vi "Read Lockin Parameters.vi"(0 "tdms file":refnum<k34>, 5 "group name in":string, 9 "Channel name":string, 11 "Error In":errorcluster, 12 "Lockin parameters":T1={"Frequency"=0.0, "Phase"=0.0, "Syncronous"=FALSE, "Points per sine wave"=0, "DDS"=FALSE, "Frequency word"=0, "Phase word"=0, "DDS modulus"=15120, "DDS clock"=125000000.0} {"DDS clock" format="%_17pHz"; "DDS modulus" format="0x%x (%d)"; "Phase" format="%#_gdeg"; "Frequency" format="%_17pHz"}) -> (2 "dt":dbl, 3 "found":bool, 4 "tdms file out":refnum<k34>, 8 "t0":timestamp, 10 "Channel length":u64, 14 "Lockin parameters out":T1={"Frequency"=0.0, "Phase"=0.0, "Syncronous"=FALSE, "Points per sine wave"=0, "DDS"=FALSE, "Frequency word"=0, "Phase word"=0, "DDS modulus"=15120, "DDS clock"=125000000.0} {"DDS clock" format="%_17pHz"; "DDS modulus" format="0x%x (%d)"; "Phase" format="%#_gdeg"; "Frequency" format="%_17pHz"}, 15 "Error Out":errorcluster)   [LabVIEW 2021]
uses:
  Lockin Parameters.ctl
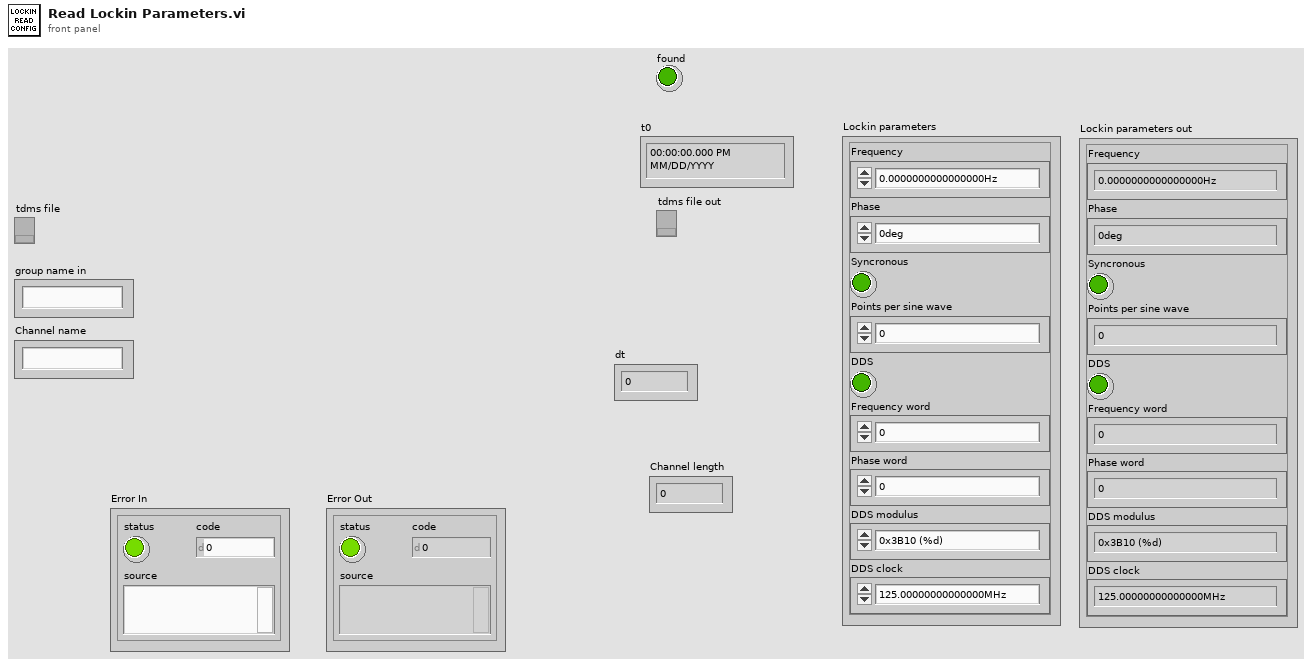
[diagram p1: front panel]
types:
  T1 = typedef "Lockin Parameters.ctl" = cluster{"Frequency":dbl, "Phase":dbl, "Syncronous":bool, "Points per sine wave":i32, "DDS":bool, "Frequency word":u32, "Phase word":u32, "DDS modulus":i64, "DDS clock":dbl}
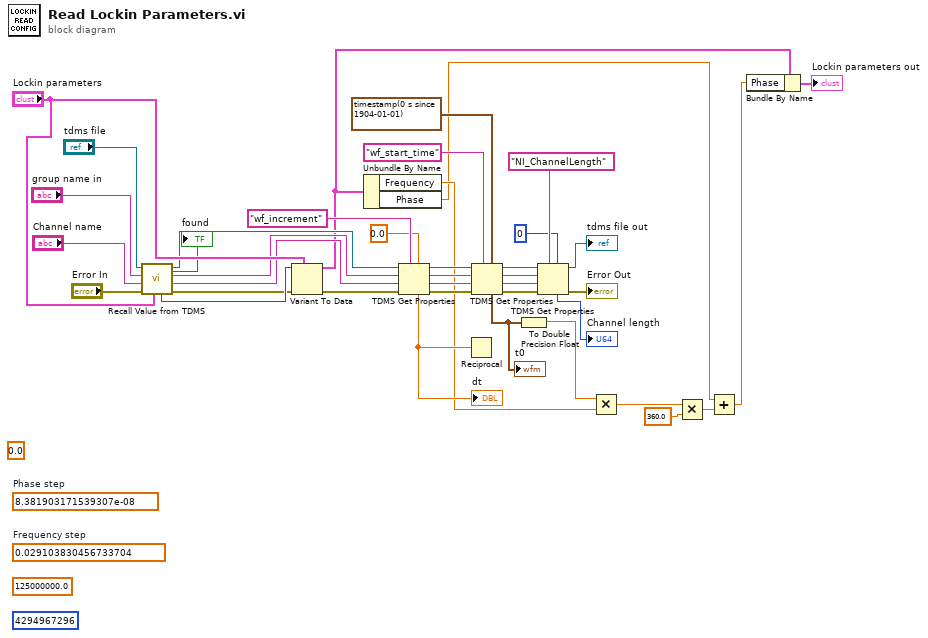
[diagram p0: block diagram]
diagram:
  (unwired) 0.0 ("index")
  (unwired) 8.381903171539307e-08  # Phase step
  (unwired) 0.029103830456733704  # Frequency step
  (unwired) u64 4294967296
  (unwired) 125000000.0
  n1 = call "Recall Value from TDMS.vi"("Value"="Lockin parameters", "Error In"="Error In", "channel name"="Channel name", "group name"="group name in", "tdms file"="tdms file") -> ("Error Out"=w24:errorcluster, "channel name out"=w16:string, "group name out"=w17:string, "tdms file out"=w22:refnum<k34>, "Value out"=w26:variant, "found"=→"found":bool)  [unwired: 1 in]
  n2 = Variant To Data(error in=w24, type="Lockin parameters", Variant=w26) -> (data=w15:T1, error out=w18:errorcluster)
  n3 = Unbundle By Name(w15) -> ("Frequency"=w14:dbl, "Phase"=w13:dbl)
  n4 = TDMS Get Properties(5:0.0, 7:"wf_increment", 8:w18, 9:w16, 10:w17, 11:w22) -> (0:w38:errorcluster, 1:w35:string, 2:w36:string, 3:w37:refnum<k34>, 4:w31:dbl)  [unwired: 1 out]
  "dt" <- w31
  n5 = Reciprocal(x=w31) -> ()  [unwired: 1 out]
  n6 = TDMS Get Properties(5:timestamp(0 s since 1904-01-01) ("t0"), 7:"wf_start_time", 8:w38, 9:w35, 10:w36, 11:w37) -> (0:w4:errorcluster, 1:w5:string, 2:w6:string, 3:w8:refnum<k34>, 4:w32:timestamp)  [unwired: 1 out]
  "t0" <- w32
  n7 = To Double Precision Float(number=w32) -> (double precision float=w30:dbl)
  n8 = TDMS Get Properties(5:u64 0, 7:"NI_ChannelLength" ("property name"), 8:w4, 9:w5, 10:w6, 11:w8) -> (0:→"Error Out":errorcluster, 3:→"tdms file out":refnum<k34>, 4:→"Channel length":u64)  [unwired: 3 out]
  n9 = Multiply(x=w30, y=w14) -> (x*y=w28:dbl)
  n10 = Multiply(x=w28, y=360.0) -> (x*y=w27:dbl)
  n11 = Add(x=w13, y=w27) -> (x+y=w11:dbl)
  n12 = Bundle By Name(cluster=w15, "Phase"=w11) -> (→"Lockin parameters out":T1)
